vi "Read Item Details.vi"(8 "error in (no error)":errorcluster, 11 "Order Item in":refnum<class "Order Item.lvclass">) -> (0 "error out":errorcluster, 2 "Description":string, 3 "Order Item out":refnum<class "Order Item.lvclass">)   [LabVIEW 2020, in "Order Item.lvclass"]
doc: "Return beverage details as a string <b>Description</b>."
uses:
  Order Item.lvclass
  Order Item.lvclass/Order Item.ctl
  Beverages/Beverage/Beverage.lvclass
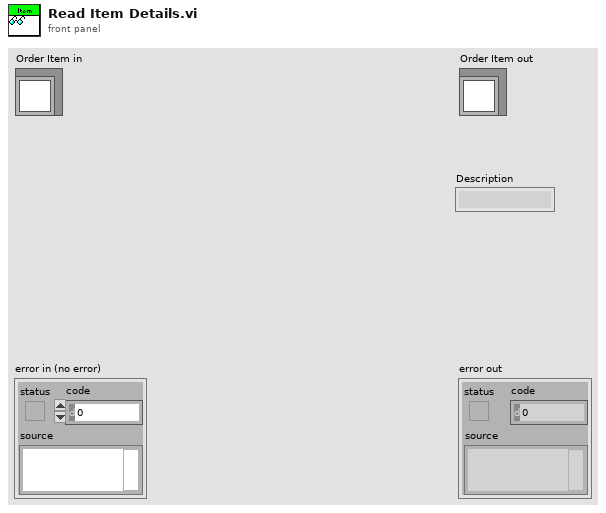
[diagram p1: front panel]
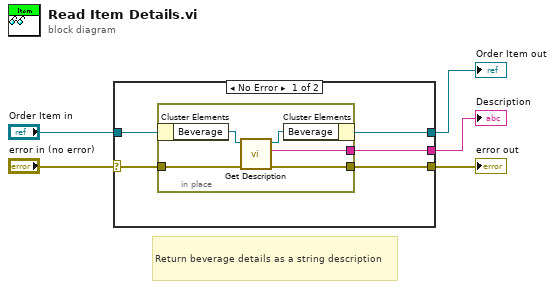
[diagram p0: block diagram]
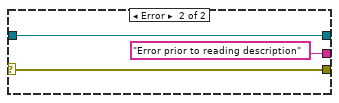
[diagram p2: hidden frame]
diagram:
  # "Return beverage details as a string description"
  n1 = case shown="No Error" "error in (no error)" {
    selector: "error in (no error)" -> [w9 w18]
    tunnel: [w8 w18] -> w4
    tunnel: [w6 w17] -> w2
    tunnel: "Order Item in" -> [w7 w17]
    tunnel: [w10 "Error prior to reading description" ("Description")] -> w1
    frame No Error {
      n2 = in-place "In Place Element Structure" {
        in-place-border: [w15] -> w10
        in-place-border: w9 -> [w14]
        in-place-border: [w13] -> w8
        n3 = in-place-cluster #1 ("Unbundle / Bundle Elements")(w7) -> ("Beverage"=w12:refnum<class "Beverage.lvclass">)
        n4 = call "Get Description.vi"("error in"=w14, "Beverage in"=w12) -> ("error out"=w13:errorcluster, "Description"=w15:string, "Beverage out"=w11:refnum<class "Beverage.lvclass">)  [unwired: 7 in]
        n5 = in-place-cluster #1 ("Unbundle / Bundle Elements")("Beverage"=w11) -> (w6:refnum<class "Order Item.lvclass">)
      }
    }
    frame Error {
    }
  }
  "error out" <- w4
  "Order Item out" <- w2
  "Description" <- w1
